vi "Add Terminal Status Channel.vi"(8 "error in":errorcluster, 11 "terminal in":T1 format="%.0x") -> (0 "error out":errorcluster, 2 "status channel":T1 format="%.0x", 3 "terminal out":T1 format="%.0x")   [LabVIEW 2020, in "Ballard MIL-STD-1553 Scripting.lvlib"]
uses:
  Ballard MIL-STD-1553 Scripting.lvlib
  <vilib>/NI VeriStand/Custom Device API/Custom Device Item Ref.ctl
  <vilib>/NI VeriStand/Custom Device API/Custom Device Channel.ctl
  <vilib>/NI VeriStand/Custom Device API/Custom Device Channel Type.ctl
  Constants.vi
  <vilib>/NI VeriStand/Custom Device API/Custom Device API.lvlib
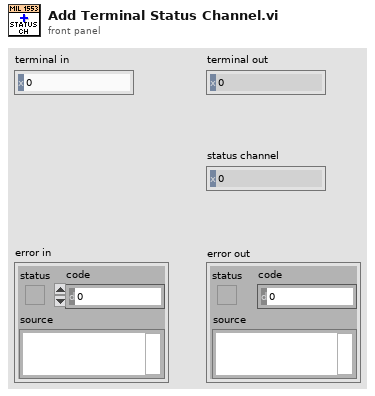
[diagram p1: front panel]
types:
  T1 = typedef "Custom Device API.lvlib/Custom Device Item Ref.ctl" = u64
  T2 = typedef "Custom Device API.lvlib/Custom Device Channel.ctl" = cluster{"Type":T3, "Units":string, "Default Value":dbl, "Faultable":bool, "Scalable":bool}
  T3 = typedef "Custom Device API.lvlib/Custom Device Channel Type.ctl" = enum16{"Input", "Output"}
  T4 = typedef "Address.ctl" = u16
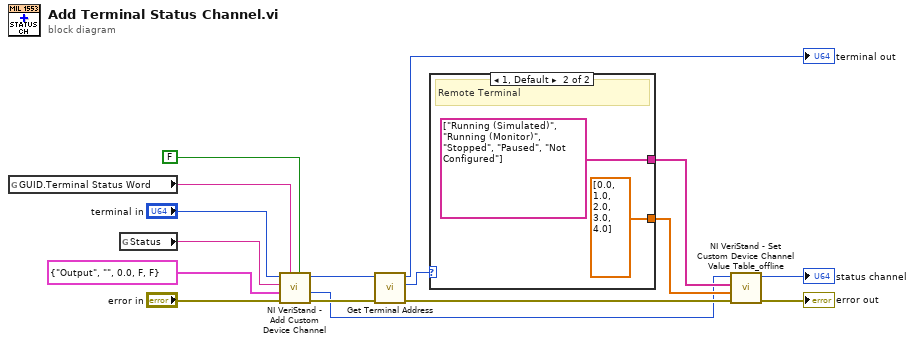
[diagram p0: block diagram]
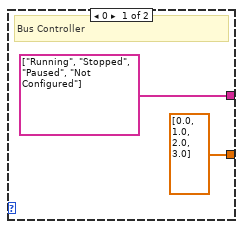
[diagram p2: hidden frame]
diagram:
  n1 = global read "Constants.vi" "GUID.Terminal Status Word"() -> (w12:string)
  n2 = global read "Constants.vi" "Status"() -> (w11:string)
  n3 = call <vilib>:"NI VeriStand - Add Custom Device Channel.vi"("Highlight? (F)"=FALSE, "GUID (Default Channel)"=w12, "error in (no error)"="error in", "Channel"=T2 {"Type"=enum."Output", "Units"="", "Default Value"=0.0, "Faultable"=FALSE, "Scalable"=FALSE}, "Channel Name"=w11, "Parent Ref in"="terminal in") -> ("error out"=w10:errorcluster, "Channel Ref"=w1:T1, "Parent Ref out"=w9:T1)  [unwired: 2 in, 1 out]
  n4 = call "Get Terminal Address.vi"("error in"=w10, "remote terminal in"=w9) -> ("error out"=w6:errorcluster, "terminal address"=w5:T4, "remote terminal out"=→"terminal out":T1)  [unwired: 6 in, 1 out]
  n5 = case shown="1, Default" w5 {
    tunnel: [dbl[] [0.0, 1.0, 2.0, 3.0] ("BC values") dbl[] [0.0, 1.0, 2.0, 3.0, 4.0] ("RT values")] -> w4
    tunnel: [string[] ["Running", "Stopped", "Paused", "Not Configured"] ("BC names") string[] ["Running (Simulated)", "Running (Monitor)", "Stopped", "Paused", "Not Configured"] ("RT names")] -> w3
    frame 0 {
      # "Bus Controller"
    }
    frame 1, Default {
      # "Remote Terminal"
    }
  }
  n6 = call "NI VeriStand - Set Custom Device Channel Value Table_offline.vi"("error in (no error)"=w6, "Values"=w4, "Names"=w3, "Channel Ref in"=w1) -> ("error out"=→"error out":errorcluster, "Channel Ref out"=→"status channel":T1)  [unwired: 6 in]
